vi "AIARG-DataAcquisition_V2.vi"() -> ()   [LabVIEW 2018]
uses:
  <vilib>/Analysis/Matrix/Datatypes/RealMatrix.ctl
  <vilib>/Utility/file.llb/Write Delimited Spreadsheet (DBL).vi
  <vilib>/Analysis/Matrix/NI_Matrix.lvlib
panel:
  in  "L11":dbl
  in  "L10":dbl
  in  "L9":dbl
  in  "L8":dbl
  in  "L7":dbl
  in  "L6":dbl
  in  "L5":dbl
  in  "L4":dbl
  in  "L3":dbl
  in  "L2":dbl
  in  "L1":dbl
  out "L11":dbl[](array[numeric])
  out "L10":dbl[](array[numeric])
  out "L9":dbl[](array[numeric])
  out "L8":dbl[](array[numeric])
  out "L7":dbl[](array[numeric])
  out "L6":dbl[](array[numeric])
  out "L5":dbl[](array[numeric])
  out "L4":dbl[](array[numeric])
  out "L3":dbl[](array[numeric])
  out "L2":dbl[](array[numeric])
  out "L1":dbl[](array[numeric])
  in  "CSV Path":path
  in  "Output Matrix":T1
  out "D1 Data":dbl[](array[numeric])
  out "SF3 Data":dbl[](array[numeric])
  out "SF2 Data":dbl[](array[numeric])
  out "SF1 Data":dbl[](array[numeric])
  out "L2 Data":dbl[](array[numeric])
  out "L1 Data":dbl[](array[numeric])
  in  "Collect Button":bool
  out "data":dynamicdata(graph)
  out "SF3":dbl
  out "SF2":dbl
  out "SF1":dbl
  out "D1":dbl
  out "L2":dbl
  out "L1":dbl
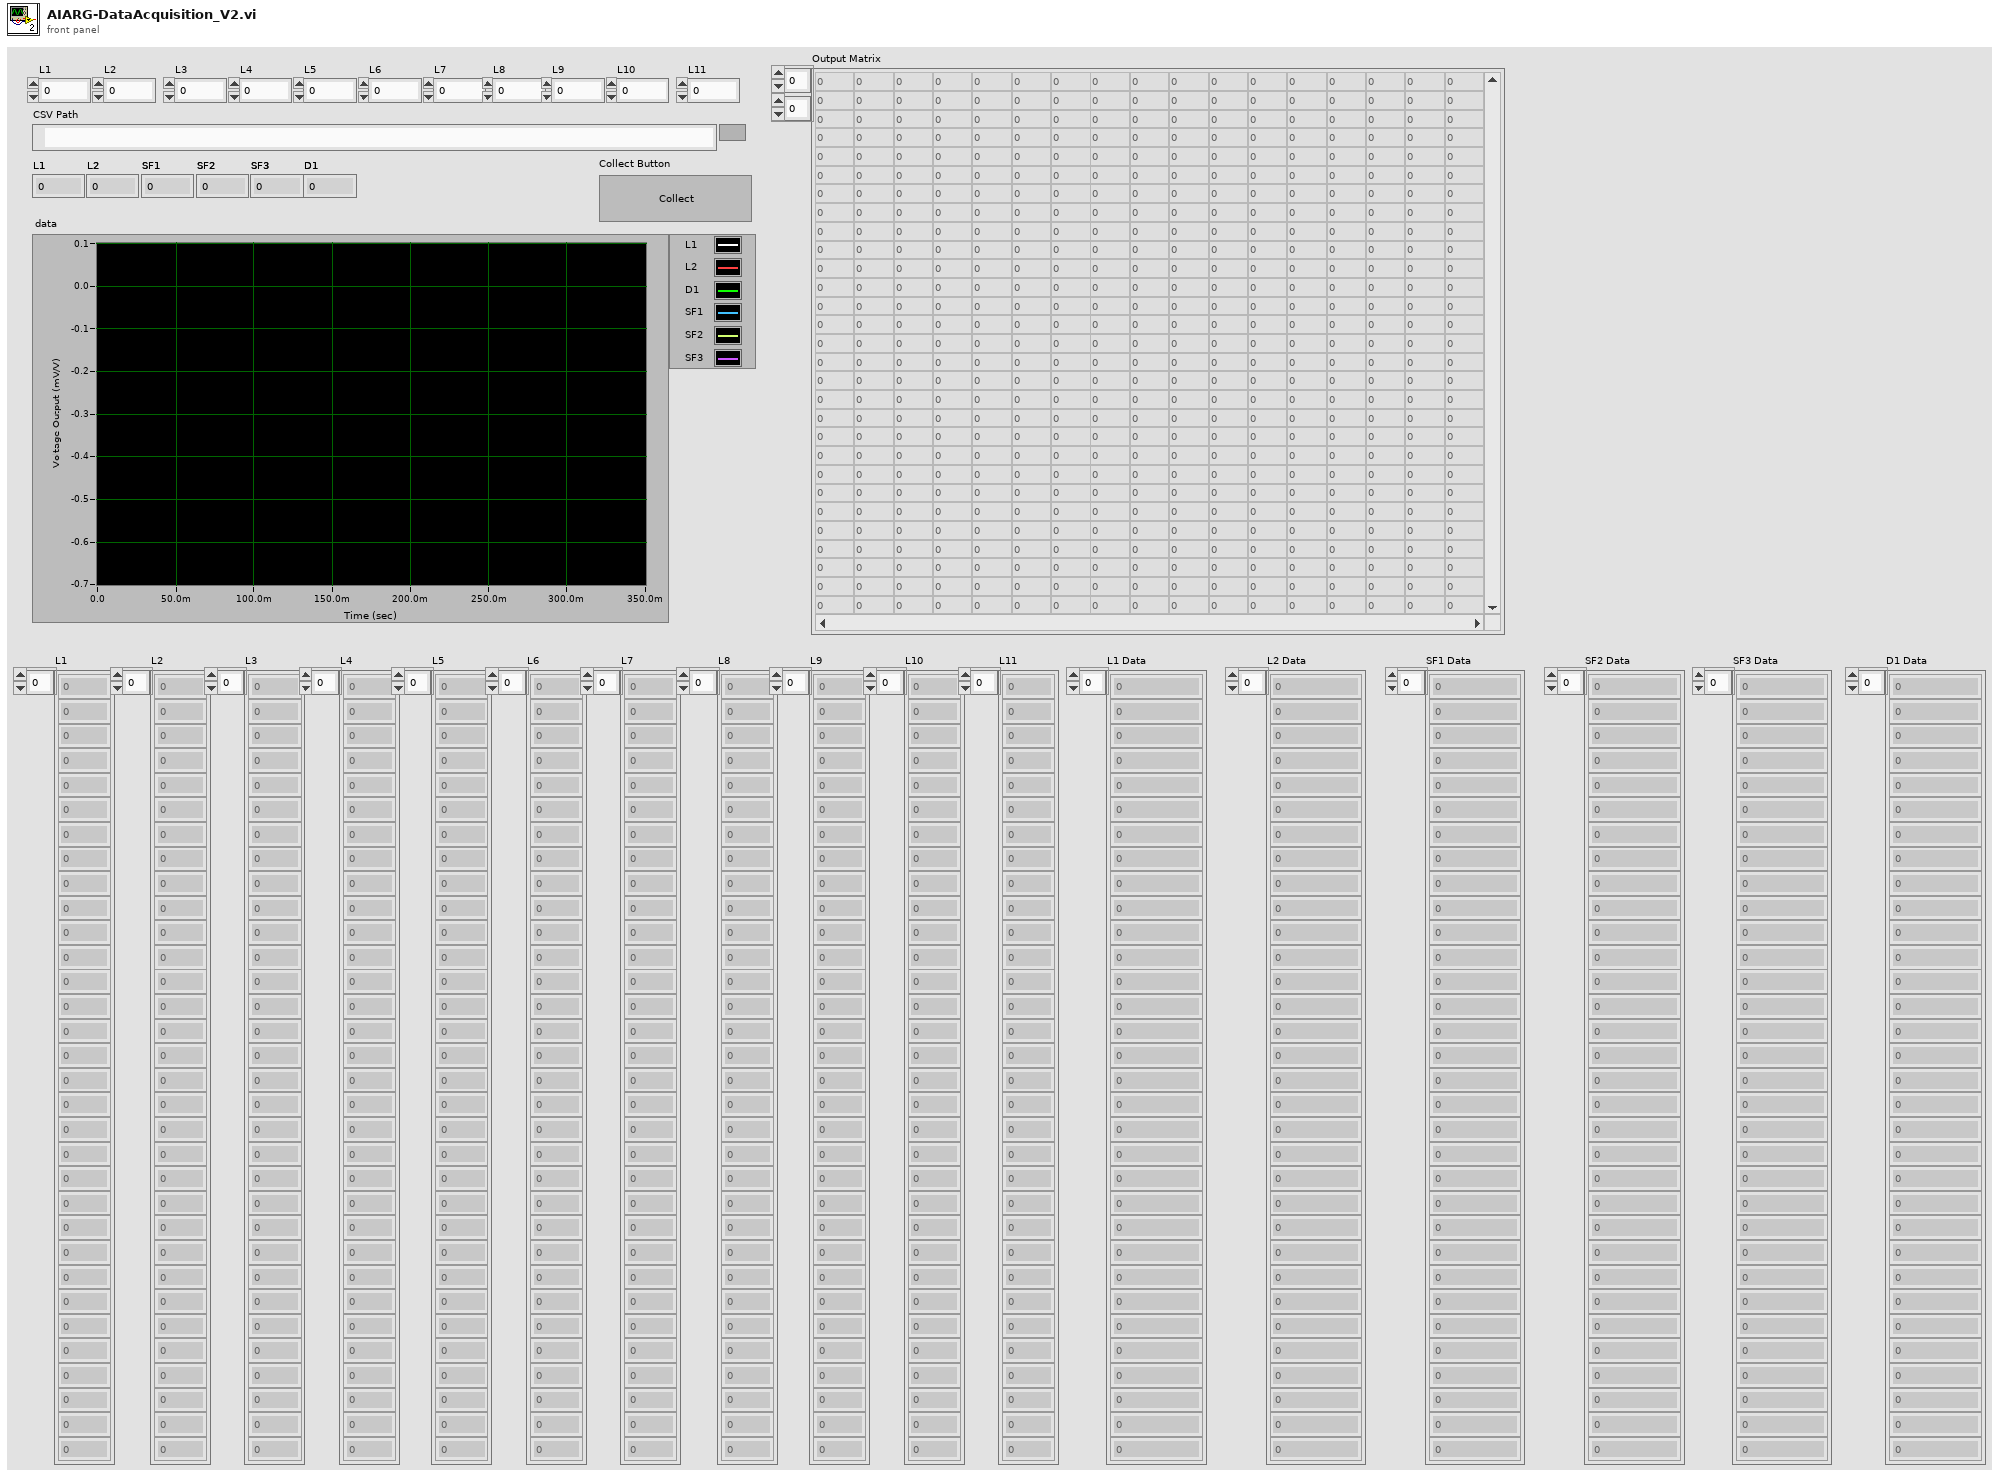
[diagram p1: front panel]
types:
  T1 = typedef "NI_Matrix.lvlib/RealMatrix.ctl" = dbl[][]
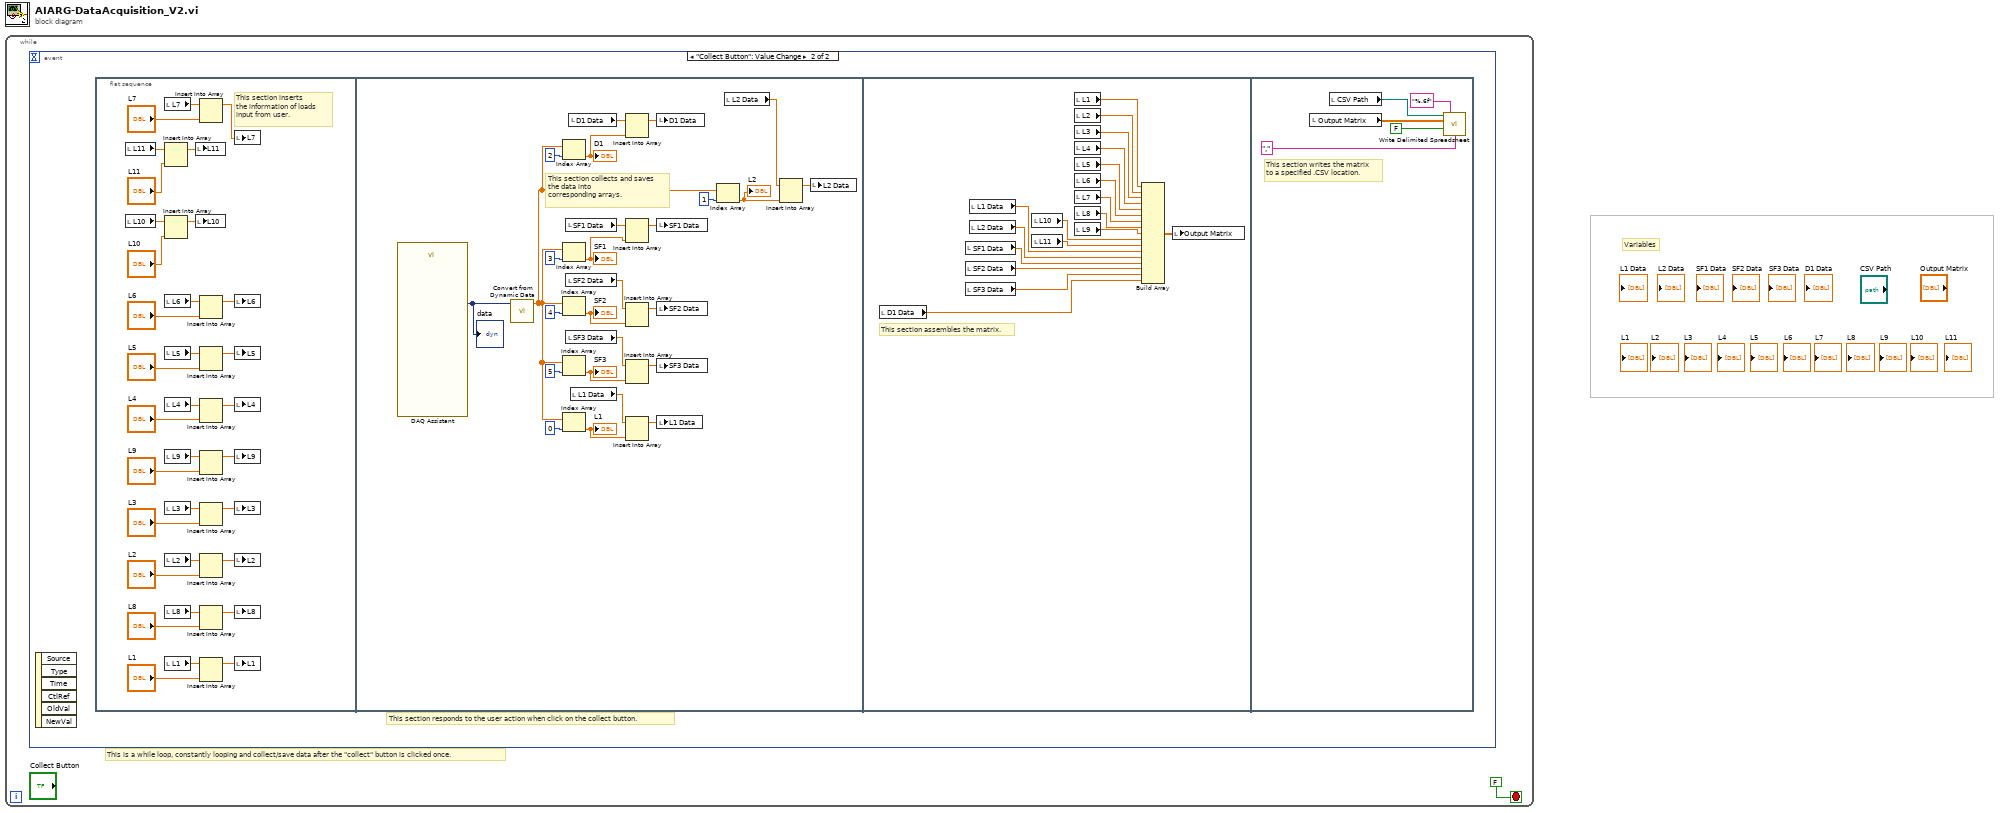
[diagram p0: block diagram]
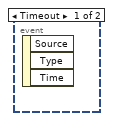
[diagram p2: hidden frame]
diagram:
  # "Variables"
  n1 = while {
    stop <- FALSE stop-if-true
    # "This is a while loop, constantly looping and collect/save data after the \"collect\" button is clicked once."
    n2 = event shown="[1] \"Collect Button\": Value Change" {
      selector: _ -> [_ _]
      dyn-events: _ -> [_ _]
      timeout: _ -> [_ _]
      event Timeout {
        n3 = event-data() -> ()  [unwired: 1 in, 3 out]
      }
      event "Collect Button": Value Change {
        # "This section responds to the user action when click on the collect button."
        n4 = event-data() -> ()  [unwired: 1 in, 6 out]
        n5 = flat-sequence {
          frame #0 {
            # "This section inserts\nthe information of loads\ninput from user."
            n6 = local read "L11"() -> (w4:dbl[])
            n7 = local read "L10"() -> (w7:dbl[])
            n8 = local read "L7"() -> (w15:dbl[])
            n9 = Insert Into Array(array=w4, new element="L11") -> (w2:dbl[])  [unwired: 1 in]
            n10 = Insert Into Array(array=w7, new element="L10") -> (w5:dbl[])  [unwired: 1 in]
            n11 = local read "L6"() -> (w18:dbl[])
            n12 = local read "L5"() -> (w21:dbl[])
            n13 = local read "L4"() -> (w24:dbl[])
            n14 = local read "L9"() -> (w10:dbl[])
            n15 = local read "L3"() -> (w27:dbl[])
            n16 = local read "L2"() -> (w31:dbl[])
            n17 = local read "L8"() -> (w12:dbl[])
            n18 = local read "L1"() -> (w34:dbl[])
            n19 = local write "L11"(w2) -> ()
            n20 = local write "L10"(w5) -> ()
            n21 = Insert Into Array(array=w15, new element="L7") -> (w16:dbl[])  [unwired: 1 in]
            n22 = Insert Into Array(array=w18, new element="L6") -> (w19:dbl[])  [unwired: 1 in]
            n23 = Insert Into Array(array=w21, new element="L5") -> (w20:dbl[])  [unwired: 1 in]
            n24 = Insert Into Array(array=w24, new element="L4") -> (w23:dbl[])  [unwired: 1 in]
            n25 = Insert Into Array(array=w10, new element="L9") -> (w8:dbl[])  [unwired: 1 in]
            n26 = Insert Into Array(array=w27, new element="L3") -> (w26:dbl[])  [unwired: 1 in]
            n27 = Insert Into Array(array=w31, new element="L2") -> (w29:dbl[])  [unwired: 1 in]
            n28 = Insert Into Array(array=w12, new element="L8") -> (w11:dbl[])  [unwired: 1 in]
            n29 = Insert Into Array(array=w34, new element="L1") -> (w32:dbl[])  [unwired: 1 in]
            n30 = local write "L7"(w16) -> ()
            n31 = local write "L6"(w19) -> ()
            n32 = local write "L5"(w20) -> ()
            n33 = local write "L4"(w23) -> ()
            n34 = local write "L9"(w8) -> ()
            n35 = local write "L3"(w26) -> ()
            n36 = local write "L2"(w29) -> ()
            n37 = local write "L8"(w11) -> ()
            n38 = local write "L1"(w32) -> ()
          }
          frame #1 {
            # "This section collects and saves \nthe data into \ncorresponding arrays."
            n39 = call "DAQ Assistant"() -> ("data"=w59:dynamicdata)  [unwired: 17 in, 2 out]
            "data" <- w59
            n40 = call "Convert from Dynamic Data"("Dynamic Data Type"=w59) -> ("Array"=w60:dbl[])  [unwired: 3 in]
            n41 = Index Array(array=w60, index=2) -> (element=w45:dbl)
            "D1" <- w45
            n42 = Index Array(array=w60, index=3) -> (element=w43:dbl)
            "SF1" <- w43
            n43 = Index Array(array=w60, index=4) -> (element=w39:dbl)
            "SF2" <- w39
            n44 = Index Array(array=w60, index=5) -> (element=w36:dbl)
            "SF3" <- w36
            n45 = Index Array(array=w60, index=0) -> (element=w51:dbl)
            "L1" <- w51
            n46 = local read "SF1 Data"() -> (w42:dbl[])
            n47 = local read "SF2 Data"() -> (w40:dbl[])
            n48 = local read "SF3 Data"() -> (w37:dbl[])
            n49 = local read "D1 Data"() -> (w46:dbl[])
            n50 = local read "L1 Data"() -> (w52:dbl[])
            n51 = Insert Into Array(array=w46, new element=w45) -> (w44:dbl[])  [unwired: 1 in]
            n52 = Insert Into Array(array=w42, new element=w43) -> (w41:dbl[])  [unwired: 1 in]
            n53 = Insert Into Array(array=w40, new element=w39) -> (w38:dbl[])  [unwired: 1 in]
            n54 = Insert Into Array(array=w37, new element=w36) -> (w35:dbl[])  [unwired: 1 in]
            n55 = Insert Into Array(array=w52, new element=w51) -> (w50:dbl[])  [unwired: 1 in]
            n56 = local write "D1 Data"(w44) -> ()
            n57 = local write "SF1 Data"(w41) -> ()
            n58 = local write "SF2 Data"(w38) -> ()
            n59 = local write "SF3 Data"(w35) -> ()
            n60 = local write "L1 Data"(w50) -> ()
            n61 = Index Array(array=w60, index=1) -> (element=w48:dbl)
            "L2" <- w48
            n62 = local read "L2 Data"() -> (w49:dbl[])
            n63 = Insert Into Array(array=w49, new element=w48) -> (w47:dbl[])  [unwired: 1 in]
            n64 = local write "L2 Data"(w47) -> ()
          }
          frame #2 {
            # "This section assembles the matrix."
            n65 = local read "D1 Data"() -> (w72:dbl[])
            n66 = local read "SF1 Data"() -> (w75:dbl[])
            n67 = local read "SF2 Data"() -> (w74:dbl[])
            n68 = local read "SF3 Data"() -> (w73:dbl[])
            n69 = local read "L1 Data"() -> (w77:dbl[])
            n70 = local read "L2 Data"() -> (w76:dbl[])
            n71 = local read "L10"() -> (w62:dbl[])
            n72 = local read "L11"() -> (w61:dbl[])
            n73 = local read "L1"() -> (w71:dbl[])
            n74 = local read "L2"() -> (w70:dbl[])
            n75 = local read "L3"() -> (w69:dbl[])
            n76 = local read "L4"() -> (w68:dbl[])
            n77 = local read "L5"() -> (w67:dbl[])
            n78 = local read "L6"() -> (w66:dbl[])
            n79 = local read "L7"() -> (w65:dbl[])
            n80 = local read "L8"() -> (w64:dbl[])
            n81 = local read "L9"() -> (w63:dbl[])
            n82 = Build Array(w71, w70, w69, w68, w67, w66, w65, w64, w63, w62, w61, w77, w76, w75, w74, w73, w72) -> (w78:dbl[][])
            n83 = local write "Output Matrix"(w78) -> ()
          }
          frame #3 {
            # "This section writes the matrix \nto a specified .CSV location."
            n84 = local read "Output Matrix"() -> (w79:T1)
            n85 = local read "CSV Path"() -> (w83:path)
            n86 = call-poly <vilib>:"Write Delimited Spreadsheet.vi"("file path (dialog if empty)"=w83, "format (%.3f)"="%.6f", "2D data"=w79, "append to file? (new file:F)"=FALSE, "delimiter (\\t)"="," ("delimiter (\\t)")) -> ()  [unwired: 9 in, 2 out]
          }
        }
      }
    }
  }
